vi "PWM Write Duty.vi"(7 "GPIO #":T1=-1, 8 "error in (no error)":errorcluster, 10 "Duty % (0-1)":sgl, 11 "Session in":refnum<class "Session.lvclass">) -> (0 "error out":errorcluster, 3 "Session out":refnum<class "Session.lvclass">)   [LabVIEW 2024, in "CTI.lvlib" / "Session.lvclass"]
doc: "Sets the duty cycle (as a range from 0.0 to 1.0) of the PWM output. The duty cycle value represents the ratio of the high portion of the PWM cycle to the low portion of the cycle. e.g. a duty cycle of 0.75 means the output will be high for 75% of the cycle."
uses:
  Session.lvclass
  GPIO Number.ctl
  DeviceComms/DeviceComms.lvclass
  CTI.lvlib
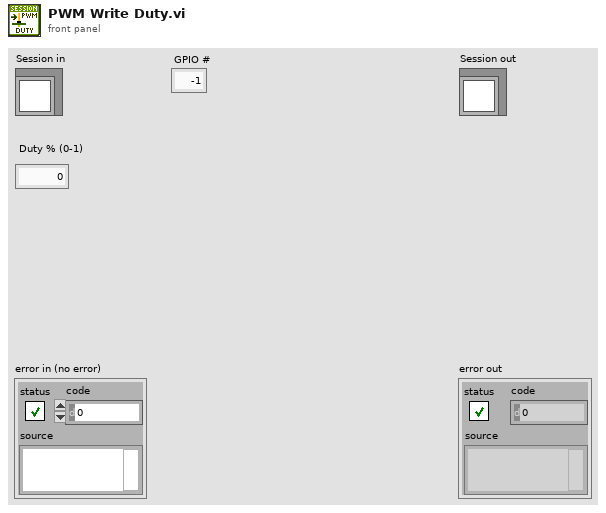
[diagram p1: front panel]
types:
  T1 = typedef "CTI.lvlib/GPIO Number.ctl" = i8
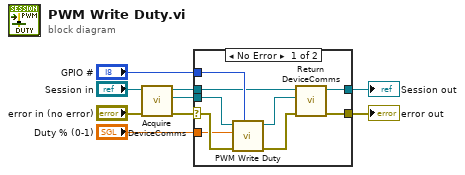
[diagram p0: block diagram]
diagram:
  n1 = call "Acquire DeviceComms.vi"("error in (no error)"="error in (no error)", "Session in"="Session in") -> ("error out"=w6:errorcluster, "DeviceComms"=w5:refnum<class "DeviceComms.lvclass">, "Session out"=w7:refnum<class "Session.lvclass">)  [unwired: 7 in]
  n2 = case shown="No Error" w6 {
    selector: w6 -> [w18 w19]
    tunnel: w7 -> [w14 w20]
    tunnel: w5 -> [w17 _]
    tunnel: "GPIO #" -> [w16 _]
    tunnel: "Duty % (0-1)" -> [w15 _]
    tunnel: [w11 w19] -> w2
    tunnel: [w10 w20] -> w1
    frame No Error {
      n3 = call-dynamic "PWM Write Duty.vi"("GPIO #"=w16, "error in (no error)"=w18, "Duty % (0-1)"=w15, "DeviceComms in"=w17) -> ("error out"=w12:errorcluster, "DeviceComms out"=w13:refnum<class "DeviceComms.lvclass">)  [unwired: 6 in]
      n4 = call "Return DeviceComms.vi"("error in (no error)"=w12, "DeviceComms"=w13, "Session in"=w14) -> ("error out"=w11:errorcluster, "Session out"=w10:refnum<class "Session.lvclass">)  [unwired: 7 in]
    }
    frame Error {
    }
  }
  "error out" <- w2
  "Session out" <- w1
